vi "Vision Processor_nocopy.vi"(7 "Image In":T2) -> (0 "error out":errorcluster, 3 "Image Out":T2(plugin-control))   [LabVIEW 2013]
uses:
  <vilib>/vision/NI_Vision_Development_Module.lvlib
  <vilib>/vision/Image Controls.llb/IMAQ Image.ctl
panel:
  out "Waveform Graph":T1(graph)
  out "Hull  Image 3":T2(plugin-control)
  out "Hull  Image 2":T2(plugin-control)
  out "Pre-Copy Image":T2(plugin-control)
  out "Processed":T2(plugin-control)
  in  "Red or Hue Range":cluster{"Lower value":i32, "Upper value":i32}={"Lower value"=0, "Upper value"=40}
  in  "Blue or Luma or Val or Inten Range":cluster{"Lower value":i32, "Upper value":i32}={"Lower value"=0, "Upper value"=47}
  in  "Green or Sat Range":cluster{"Lower value":i32, "Upper value":i32}={"Lower value"=21, "Upper value"=226}
  out "Pre-Process":T2(plugin-control)
  # "0  center of mass x\n1  center of mass y\n2  first pixel x\n3  first pixel y\n4  bounding rect left\n5  bounding rect top\n6  bounding rect right\n7  bounding rect bottom\n8 max feret diameter start x\n9  max feret diameter start y\n10 max feret diameter end x\n11 max feret diameter end y\n12 max horiz segment length left\n13 max horiz segment length right\n14 max horiz segment length row\n15 bounding rect width \n16 bounding rect height\n17 bounding rect diagional\n..\n33 area"
  # "13'3\"\n3'9\""
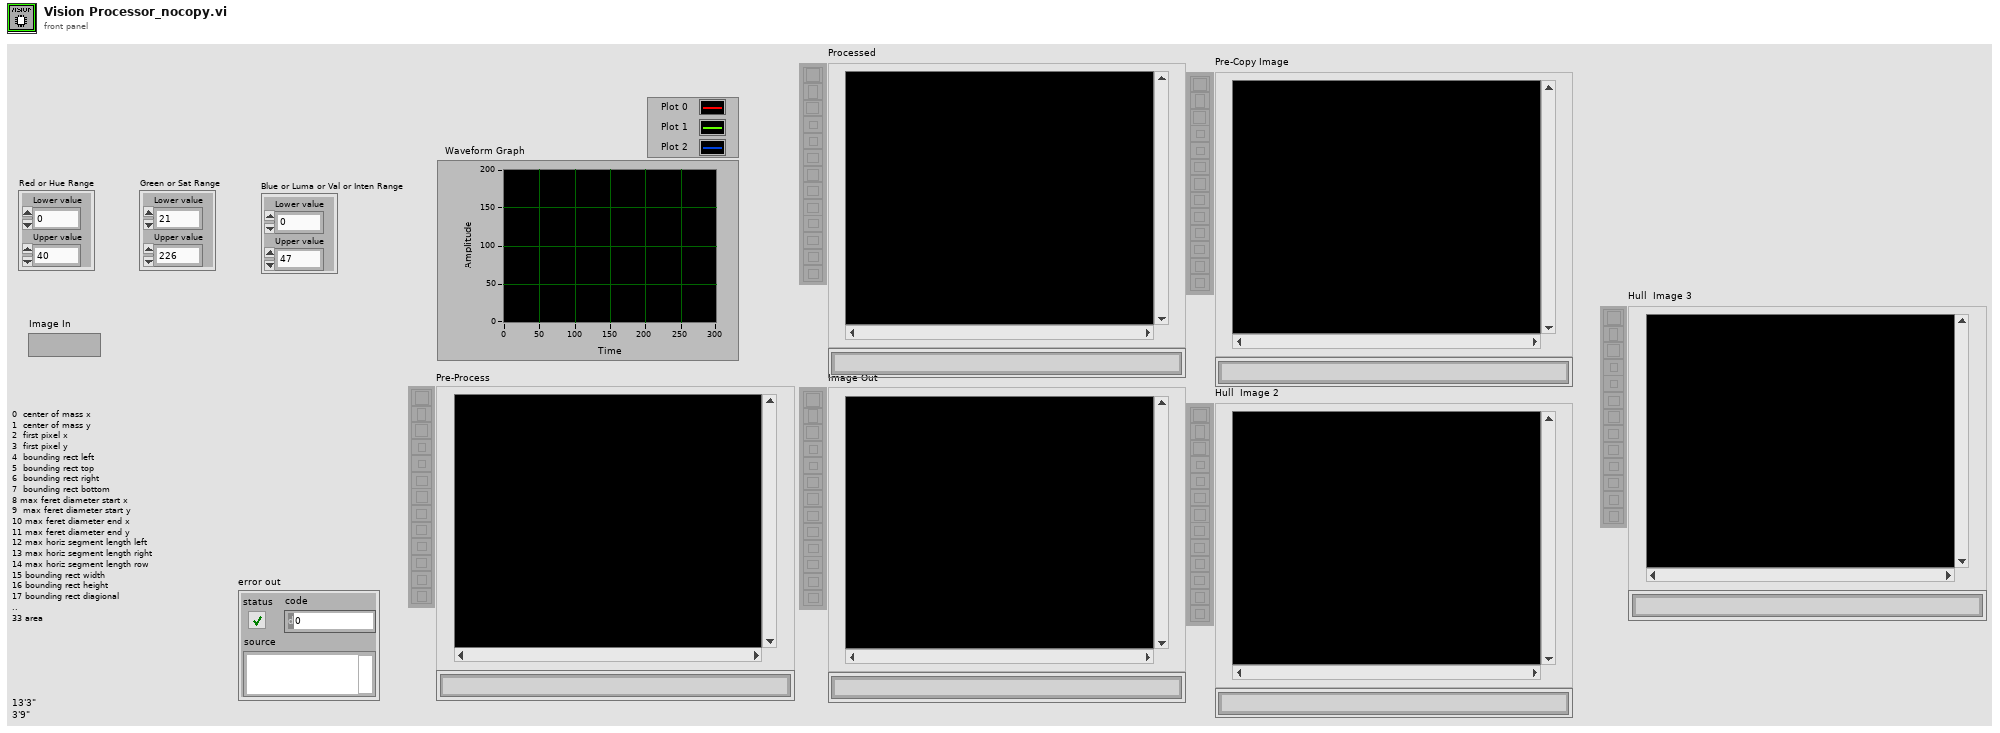
[diagram p1: front panel]
types:
  T1 = cluster{"Starting Value":sgl, "Incremental Value":sgl, "Histogram":u32[]}[]
  T2 = typedef "IMAQ Image.ctl" = refnum<image>
  T3 = typedef "Image Type" = u32
  T4 = enum32{"AutoM", "Close", "Dilate", "Erode", "Gradient", "Gradient out", "Gradient in", "Hit miss", "Open", "PClose", "POpen", "Thick", "Thin"}
  T5 = cluster{"Starting Value":sgl, "Incremental Value":sgl, "Histogram":u32[]}
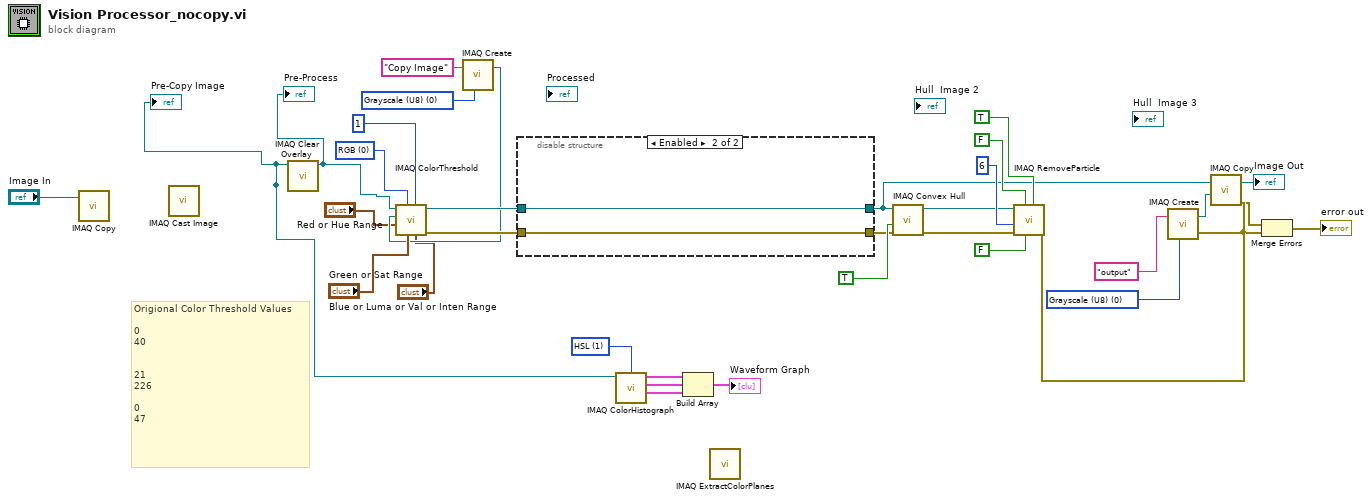
[diagram p0: block diagram]
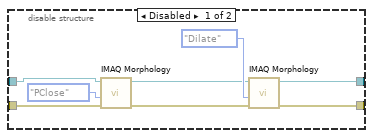
[diagram p2: hidden frame]
diagram:
  w6 = u16 1 items=["RGB", "HSL", "HSV", "HSI"] ("Color Mode")
  w15 = T3 0 items=["Grayscale (U8)", "Grayscale (I16)", "Grayscale (SGL)", "Complex (CSG)", "RGB (U32)", "HSL (U32)", "RGB (U64)", "Grayscale (U16)"] ("Image Type")
  w26 = T3 0 items=["Grayscale (U8)", "Grayscale (I16)", "Grayscale (SGL)", "Complex (CSG)", "RGB (U32)", "HSL (U32)", "RGB (U64)", "Grayscale (U16)"] ("Image Type")
  w34 = u16 0 items=["RGB", "HSL", "HSV", "HSI"] ("Color Mode")
  # "Origional Color Threshold Values\n\n0\n40\n\n\n21\n226\n\n0\n47"
  n1 = call "IMAQ Copy"("Image Src"="Image In") -> ()  [unwired: 5 in, 2 out]
  n2 = call "IMAQ Cast Image"() -> ()  [unwired: 10 in, 2 out]
  n3 = call "IMAQ Clear Overlay"("Image"="Pre-Copy Image") -> ("Image Out"=w11:T2)  [unwired: 9 in, 1 out]
  "Pre-Process" <- w11
  n4 = call "IMAQ Create"("Image Name"="Copy Image", "Image Type"=w15) -> ("New Image"=w12:T2)  [unwired: 3 in, 1 out]
  n5 = call "IMAQ ColorThreshold"("Blue or Luma or Val or Inten Range"="Blue or Luma or Val or Inten Range", "Replace Value"=1, "Green or Sat Range"="Green or Sat Range", "Color Mode"=w34, "Red or Hue Range"="Red or Hue Range", "Image Dst"=w12, "Image Src"=w11) -> ("error out"=w28:errorcluster, "Image Dst Out"=w17:T2)  [unwired: 1 in, 2 out]
  n6 = disable-structure shown="Enabled" {
    disable-tunnel: w17 -> [w42 w45]
    disable-tunnel: w28 -> [w41 w44]
    disable-tunnel: [w37 w45] -> w3
    disable-tunnel: [w36 w44] -> w23
    frame Disabled {
      n7 = call "IMAQ Morphology"("error in (no error)"=w41, "Operation"=T4."PClose", "Image Src"=w42) -> ("error out"=w39:errorcluster, "Image Dst Out"=w38:T2)  [unwired: 7 in]
      n8 = call "IMAQ Morphology"("error in (no error)"=w39, "Operation"=T4."Dilate", "Image Src"=w38) -> ("error out"=w36:errorcluster, "Image Dst Out"=w37:T2)  [unwired: 7 in]
    }
    frame Enabled {
    }
  }
  n9 = call "IMAQ ColorHistograph"("Color Mode"=w6, "Image Src"="Pre-Copy Image") -> ("Red or Hue Histogram Graph"=w10:T5, "Green or Sat Histogram Graph"=w9:T5, "Blue or Luma or Val or Inten Histogram Graph"=w8:T5)  [unwired: 4 in, 1 out]
  n10 = Build Array(w10, w9, w8) -> (→"Waveform Graph":T1)
  n11 = call "IMAQ ExtractColorPlanes"() -> ()  [unwired: 8 in, 4 out]
  n12 = call "IMAQ Convex Hull"("error in (no error)"=w23, "Connectivity 4/8 (8)"=TRUE, "Image Src"=w3) -> ("error out"=w27:errorcluster, "Image Dst Out"=w13:T2)  [unwired: 1 in, 6 out]
  n13 = call "IMAQ RemoveParticle"("Connectivity 4/8 (8)"=TRUE, "Low Pass/High Pass (Low)"=FALSE, "Square/Hexa (Square)"=FALSE, "error in (no error)"=w27, "Number of Erosion"=6, "Image Src"=w13) -> ("error out"=w21:errorcluster)  [unwired: 1 in, 4 out]
  n14 = call "IMAQ Create"("Image Name"="output", "Image Type"=w26, "error in (no error)"=w21) -> ("New Image"=w24:T2, "error out"=w20:errorcluster)  [unwired: 2 in]
  n15 = call "IMAQ Copy"("error in (no error)"=w21, "Image Dst"=w24, "Image Src"=w3) -> ("error out"=w19:errorcluster, "Image Dst Out"=→"Image Out":T2)  [unwired: 3 in]
  n16 = Merge Errors(w19, w20) -> (→"error out":errorcluster)
